vi "scale to u8.vi"(11 "Input":sgl[](array[numeric])) -> (3 "Output":sgl[](array[numeric]))   [LabVIEW 2013]
uses:
  <vilib>/Analysis/NI_AALPro.lvlib
panel:
  out "10% min value":sgl
  out "old min value":sgl
  out "old max value":sgl
  out "new histogam":T1(graph)
  out "Histogram Graph":T1(graph)
  out "10% max value":sgl
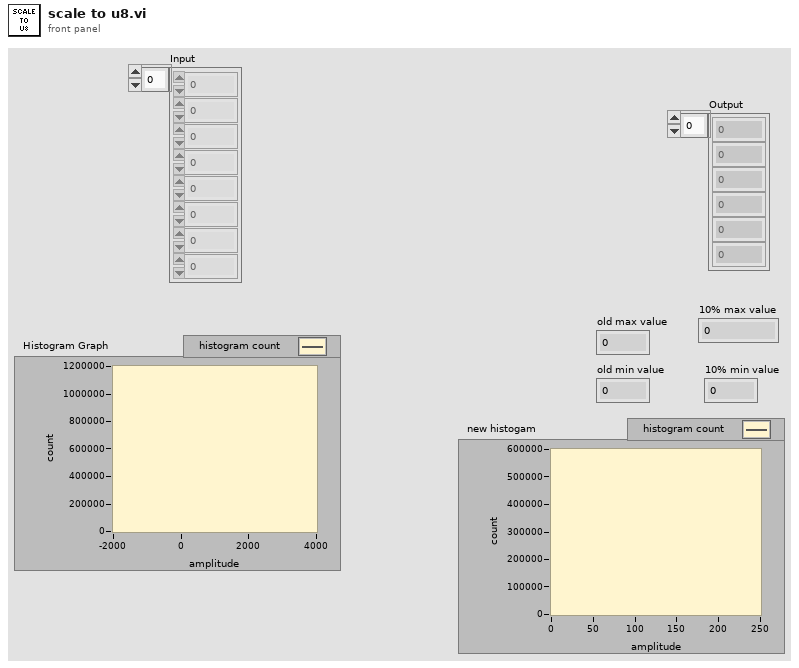
[diagram p1: front panel]
types:
  T1 = cluster{"X Values":dbl[], "Histogram: h(x)":i32[]}
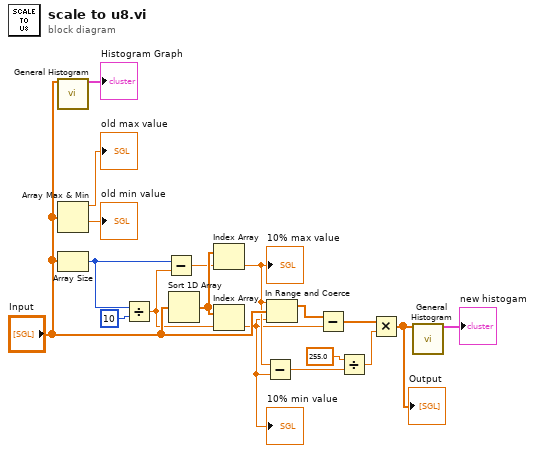
[diagram p0: block diagram]
diagram:
  n1 = call <vilib>:"General Histogram.vi"("X"="Input") -> ("Histogram Graph"=→"Histogram Graph":T1)  [unwired: 10 in, 4 out]
  n2 = Array Max & Min(array="Input") -> (max value=→"old max value":sgl, min value=→"old min value":sgl)  [unwired: 2 out]
  n3 = Array Size(array="Input") -> (size(s)=w5:i32)
  n4 = Divide(x=w5, y=10) -> (x/y=w4:dbl)
  n5 = Subtract(x=w5, y=w4) -> (x-y=w3:dbl)
  n6 = Sort 1D Array(array="Input") -> (sorted array=w6:sgl[])
  n7 = Index Array(array=w6, index=w3) -> (element=w2:sgl)
  "10% max value" <- w2
  n8 = Index Array(array=w6, index=w4) -> (element=w1:sgl)
  "10% min value" <- w1
  n9 = Subtract(x=w2, y=w1) -> (x-y=w12:sgl)
  n10 = In Range and Coerce(upper limit=w2, x="Input", lower limit=w1) -> (coerced(x)=w13:sgl[])  [unwired: 1 out]
  n11 = Subtract(x=w13, y=w1) -> (x-y=w10:sgl[])
  n12 = Divide(x=sgl 255.0, y=w12) -> (x/y=w9:sgl)
  n13 = Multiply(x=w10, y=w9) -> (x*y=w8:sgl[])
  "Output" <- w8
  n14 = call <vilib>:"General Histogram.vi"("X"=w8) -> ("Histogram Graph"=→"new histogam":T1)  [unwired: 10 in, 4 out]
